vi "Copy from XY graph.vi"(8 "error in (no error)":errorcluster, 9 "ItemTag":string, 10 "Type of graph":string(combo)="Kinetics", 11 "Control-Client in":refnum<class "Control-Client.lvclass">) -> (0 "error out":errorcluster, 3 "Control-Client out":refnum<class "Control-Client.lvclass">)   [LabVIEW 2018, in "Control-Client.lvclass"]
uses:
  Control-Client.lvclass
  Control-Client.lvclass/Control-Client.ctl
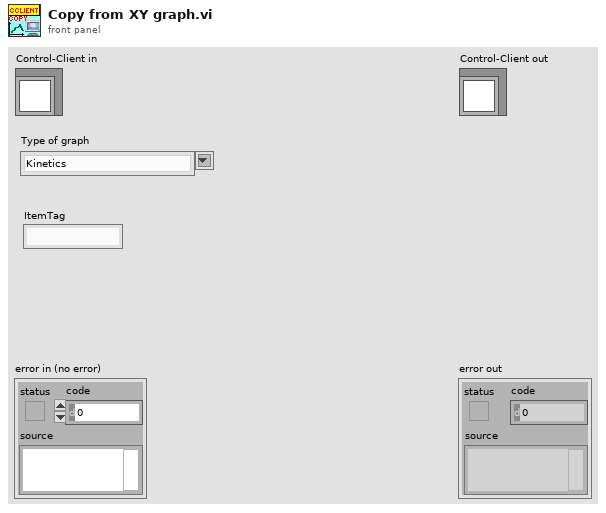
[diagram p1: front panel]
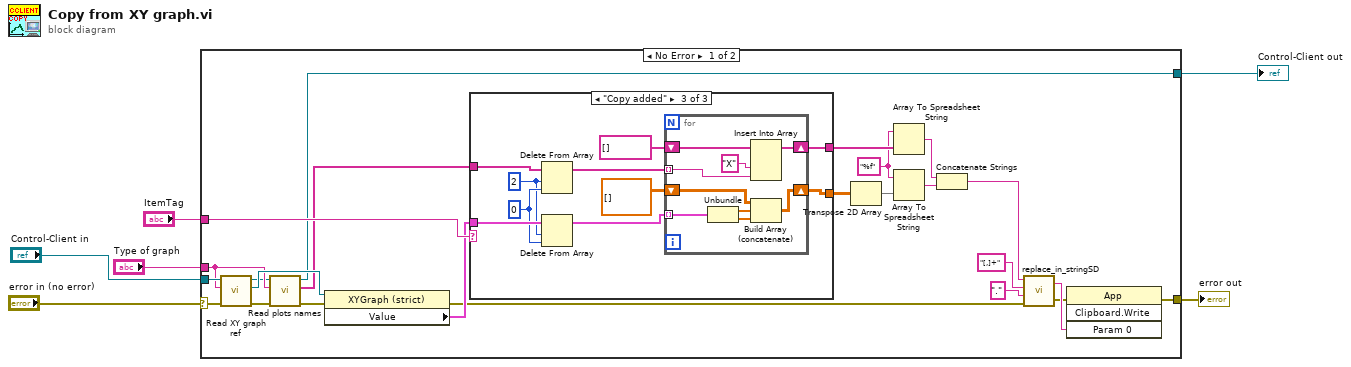
[diagram p0: block diagram]
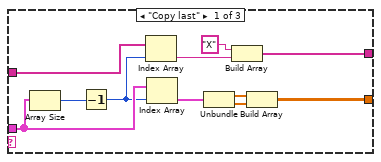
[diagram p2: hidden frame]
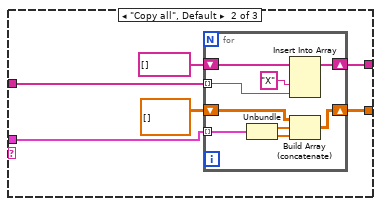
[diagram p3: hidden frame]
diagram:
  n1 = case shown="No Error" "error in (no error)" {
    selector: "error in (no error)" -> [w23 w77]
    tunnel: [w25 w77] -> w5
    tunnel: [w7 w76] -> w3
    tunnel: "Control-Client in" -> [w18 w76]
    tunnel: "ItemTag" -> [w24 _]
    tunnel: "Type of graph" -> [w17 _]
    frame No Error {
      w9 = "%f" ("format string")
      n2 = call "Read XY graph ref.vi"("error in (no error)"=w23, "Combo Box"=w17, "Control-Client in"=w18) -> ("error out"=w15:errorcluster, "XY graph ref"=w21:refnum<vi>, "Control-Client out"=w16:refnum<class "Control-Client.lvclass">)  [unwired: 6 in]
      n3 = call "Read plots names.vi"("error in (no error)"=w15, "Combo Box"=w17, "Control-Client in"=w16) -> ("error out"=w14:errorcluster, "Plots names"=w13:string[], "Control-Client out"=w7:refnum<class "Control-Client.lvclass">)  [unwired: 6 in]
      n4 = property class="XYGraph (strict)"(reference=w21, error in=w14) -> (error out=w19:errorcluster, "Value"=w20:cluster{"Y":dbl[], "Y":dbl[]}[])  [unwired: 1 out]
      n5 = case shown="\"Copy added\"" w24 {
        tunnel: [w36 w46 w65] -> w27
        tunnel: w20 -> [w38 w45 w64]
        tunnel: w13 -> [w35 w44 w62]
        tunnel: [w31 w42 w57] -> w12
        frame "Copy last" {
          n6 = Array Size(array=w38) -> (size(s)=w41:i32)
          n7 = Decrement(x=w41) -> (x-1=w34:i32)
          n8 = Index Array(array=w35, index=w34) -> (element=w33:string)
          n9 = Index Array(array=w38, index=w34) -> (element=w37:cluster{"Y":dbl[], "Y":dbl[]})
          n10 = Unbundle(w37) -> ("Y"=w40:dbl[], "Y"=w39:dbl[])
          n11 = Build Array("X" ("element"), w33) -> (w31:string[])
          n12 = Build Array(w40, w39) -> (w36:dbl[][])
        }
        frame "Copy all", Default {
          n13 = for {
            shift-right: [w52] -> w46
            shift-left: dbl[][] [] ("appended array") -> [w56]
            tunnel: w45 -> [w55] mode=indexing
            tunnel: w44 -> [w48] mode=indexing
            shift-right: [w50] -> w42
            shift-left: string[] [] ("Plots names") -> [w51]
            n14 = Unbundle(w55) -> ("Y"=w54:dbl[], "Y"=w53:dbl[])
            n15 = Insert Into Array(array=w51, new element #1="X" ("element"), new element #2=w48) -> (w50:string[])  [unwired: 1 in]
            n16 = Build Array (concatenate)(w56, w54, w53) -> (w52:dbl[][])
          }
        }
        frame "Copy added" {
          w61 = 0 ("index")
          w60 = 2 ("length")
          n17 = Delete From Array(array=w62, length=w60, index=w61) -> (array with subset deleted=w58:string[])  [unwired: 1 out]
          n18 = Delete From Array(array=w64, length=w60, index=w61) -> (array with subset deleted=w63:cluster{"Y":dbl[], "Y":dbl[]}[])  [unwired: 1 out]
          n19 = for {
            shift-right: [w71] -> w65
            shift-left: dbl[][] [] ("appended array") -> [w75]
            tunnel: w63 -> [w74] mode=indexing
            shift-right: [w69] -> w57
            shift-left: string[] [] ("Plots names") -> [w70]
            tunnel: w58 -> [w67] mode=indexing
            n20 = Unbundle(w74) -> ("Y"=w73:dbl[], "Y"=w72:dbl[])
            n21 = Insert Into Array(array=w70, new element #1="X" ("element"), new element #2=w67) -> (w69:string[])  [unwired: 1 in]
            n22 = Build Array (concatenate)(w75, w73, w72) -> (w71:dbl[][])
          }
        }
      }
      n23 = Transpose 2D Array(2D array=w27) -> (transposed array=w26:dbl[][])
      n24 = Array To Spreadsheet String(array=w12, 3:w9) -> (spreadsheet string=w11:string)  [unwired: 1 in]
      n25 = Array To Spreadsheet String(array=w26, 3:w9) -> (spreadsheet string=w10:string)  [unwired: 1 in]
      n26 = Concatenate Strings(w11, w10) -> (w8:string)
      n27 = call "replace_in_stringSD.vi"("error in (no error)"=w19, "replaced to.."=".", "characters to replace"="[,]+", "input string"=w8) -> ("error out"=w22:errorcluster, "output string"=w28:string)
      n28 = invoke class="App" method="Clipboard.Write"(error in=w22, "Param 0"=w28) -> (error out=w25:errorcluster)  [unwired: 2 in, 3 out]
    }
    frame Error {
    }
  }
  "error out" <- w5
  "Control-Client out" <- w3
